vi "Attribute to Service Details.vi"(0 "Attibute Found":bool, 3 "Attribute":variant) -> (17 "Service Enqueuer":refnum<class "Message Enqueuer.lvclass">)   [LabVIEW 2016, in "WebSocket Actors.lvlib" / "WebSocket Server.lvclass"]
uses:
  WebSocket Server.lvclass
  <vilib>/ActorFramework/Message Enqueuer/Message Enqueuer.lvclass
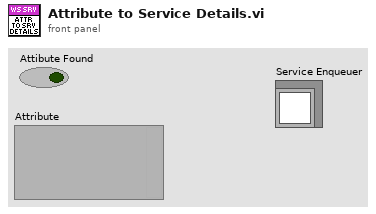
[diagram p1: front panel]
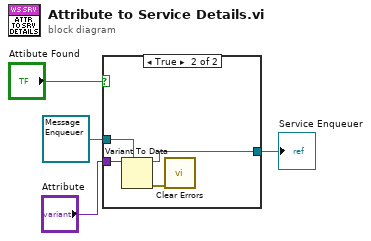
[diagram p0: block diagram]
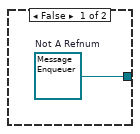
[diagram p2: hidden frame]
diagram:
  n1 = case shown="True" "Attibute Found" {
    tunnel: "Attribute" -> [_ w8]
    tunnel: [w5 w7] -> w1
    tunnel: refnum<class "Message Enqueuer.lvclass"> refnum ("Service Enqueuer") -> [_ w6]
    frame False {
      w5 = refnum<class "Message Enqueuer.lvclass"> refnum  # Not A Refnum
    }
    frame True {
      n2 = Variant To Data(type=w6, Variant=w8) -> (data=w7:refnum<class "Message Enqueuer.lvclass">, error out=w9:errorcluster)  [unwired: 1 in]
      n3 = call <vilib>:"Clear Errors.vi"("error in (no error)"=w9) -> ()  [unwired: 5 in, 2 out]
    }
  }
  "Service Enqueuer" <- w1
